vi "TermoRead.vi"() -> ()   [LabVIEW 2018]
uses:
  <vilib>/Analysis/Matrix/Datatypes/RealMatrix.ctl
  LW/Termodat_16K5/Control 2.ctl
  LW/Termodat_16K5/Control 4.ctl
  LW/Termodat_16K5/Control 3.ctl
  LW/Termodat_16K5/Control 1.ctl
  LW/Termodat_16K5/Control 5.ctl
  <instrlib>/Tektronix DMM40x0 Series/Tektronix DMM40x0 Series.lvlib
  LW/LIRA_toolbox.lvlib
  <vilib>/Analysis/Matrix/NI_Matrix.lvlib
panel:
  out "Ошибка с Modbus":errorcluster
  in  "Температура ТД":T1={"Измеряемая величина"="Ttd", "единицы измерения"="C", "Ширина строки (в символах)"="16", "Количество знаков после запятой"="2"}
  in  "Температура":T1={"Измеряемая величина"="T", "единицы измерения"="C", "Ширина строки (в символах)"="16", "Количество знаков после запятой"="2"}
  in  "Сопротивление":T1={"Измеряемая величина"="R", "единицы измерения"="Ом", "Ширина строки (в символах)"="16", "Количество знаков после запятой"="2"}
  in  "Параметры общения с Термодат":T7={"Baud Rate"=19200, "Parity"=0, "Flow Control"=0, "Timeout"=300, "Mode"=enum."RTU", "VISA resource name"="COM4", "Timeout 2"=300, "Serial Parameters"={"Mode"=enum."ASCII", "Slave Address"=1}, "Starting Address"=0, "Quantity"=1} {"Serial Parameters"."Slave Address" format="%.0x"; "Flow Control" items=["None", "XON/XOFF", "RTS/CTS", "XON/XOFF & RTS/CTS", "DTR/DSR", "XON/XOFF & DTR/DSR"]; "Parity" items=["None", "Odd", "Even", "Mark", "Space"]}
  in  "Количество датчиков Термодат":i32=2
  out "Ошибка записи в файл":errorcluster
  out "Ошибка перключения":errorcluster
  in  "Задача":refnum<k21>="Generete_Termo_Dat"
  out "T1":T8(graph)
  in  "Function (0: DC Voltage)":u16(ring)=3 items=["DC Voltage", "AC Voltage", "2 - Wire Resistance", "4 - Wire Resistance", "DC Current", "AC Current", "Frequency", "Period", "Continuity", "Diode Checking", "Temperature", "Capacitance"]
  in  "Real Matrix":T9=[[0.0, 1.0, 0.0, 0.0], [0.0, 1.0, 0.0, 0.0], [0.0, 0.0, 0.0, 1.0], [0.0, 0.0, 0.0, 1.0], [0.0, 0.0, 1.0, 1.0], [0.0, 0.0, 1.0, 1.0]]
  in  "Сопротивление при нуле":dbl=60.0
  in  "alpha":dbl=0.00428
  out "Что следует из алгоритма":bool[](array[boolean])
  out "Array":bool[][](array[boolean])
  in  "Период перключения":dbl=2.0 caption="Delay Time (s)"
  in  "Название файла":string="TempData"
  in  "Путь к файлу с указанием\n на случайный txt файл":path=path "E:/Температурные датчики/Log/20250605_19_09_TempData.txt"
  in  "Количество датчиков":i32=4
  out "Ошибка прибора":errorcluster
  out "VISA resource name out":refnum<visa-resource-name>
  out "output array":dbl[](array[numeric]) format="%^_7e"
  in  "Serial Configuration":T10={"Baud Rate"=19200, "Parity"=0, "Data Bits"=8, "Stop Bits"=10, "Flow Control"=0} {"Flow Control" items=["None", "XON/XOFF", "RTS/CTS", "XON/XOFF & RTS/CTS", "DTR/DSR", "XON/XOFF & DTR/DSR"]; "Stop Bits" items=["1.0"=10, "1.5"=15, "2.0"=20]; "Data Bits" items=["7"=7, "8"=8]; "Parity" items=["None", "Odd", "Even", "Mark", "Space"]; "Baud Rate" items=["300"=300, "600"=600, "1200"=1200, "2400"=2400, "4800"=4800, "9600"=9600, "19200"=19200]}
  in  "VISA resource name":refnum<visa-resource-name>="COM5"
  in  "stop":bool
  # "Параметры для создания log файла"
  # "Параметры для расчёта температуры"
  # "Схема включения каналов"
  # "Параметры процесса измерения"
  # "Каждая колонка соответсвует определённому датчику\nКаждый ряд соответствует определённому реле"
  # "Подключение к Tetronix DMM4040"
  # "Индикация для отадки"
  # "График температур"
  # "Параметры инициализации"
  # "Параметры чтения"
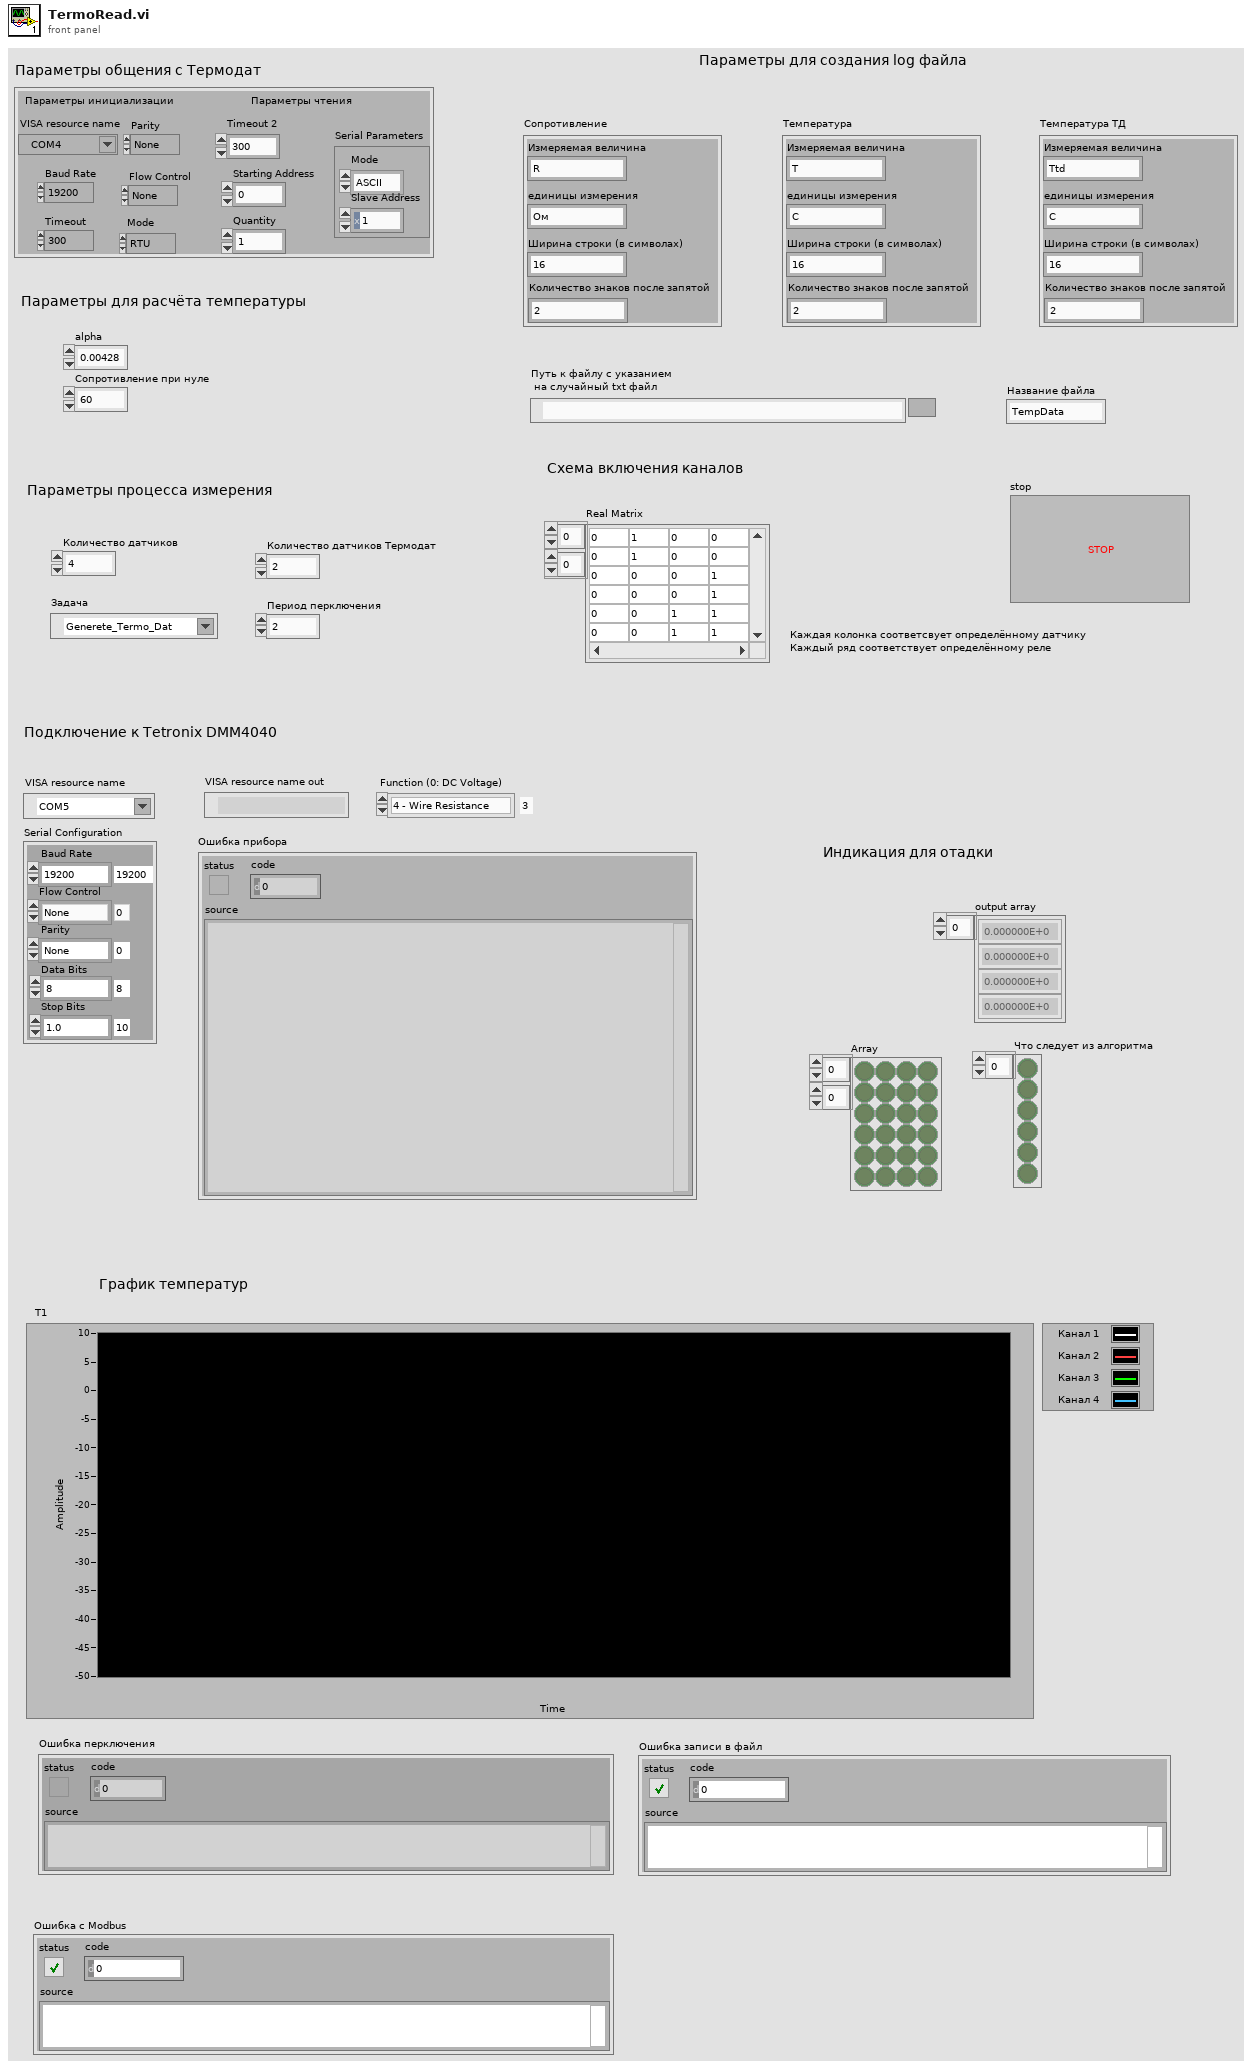
[diagram p1: front panel]
types:
  T1 = cluster{"Измеряемая величина":string, "единицы измерения":string, "Ширина строки (в символах)":string, "Количество знаков после запятой":string}
  T2 = typedef "Control 2.ctl" = u32
  T3 = typedef "Control 4.ctl" = u32
  T4 = typedef "Control 3.ctl" = enum16{"RTU", "ASCII"}
  T5 = typedef "Control 1.ctl" = refnum<visa-resource-name>
  T6 = typedef "Control 5.ctl" = u32
  T7 = cluster{"Baud Rate":T2, "Parity":u16, "Flow Control":u16, "Timeout":T3, "Mode":T4, "VISA resource name":T5, "Timeout 2":T6, "Serial Parameters":cluster{"Mode":enum16{"RTU", "ASCII"}, "Slave Address":u8}, "Starting Address":u16, "Quantity":u16}
  T8 = cluster{"Массив температур[0]":dbl, "Массив температур[1]":dbl, "Массив температур[2]":dbl, "Массив температур[3]":dbl, "Массив температур[4]":dbl, "Массив температур[5]":dbl, "Массив температур[6]":dbl, "Массив температур[7]":dbl, "Массив температур[8]":dbl}
  T9 = typedef "NI_Matrix.lvlib/RealMatrix.ctl" = dbl[][]
  T10 = cluster{"Baud Rate":u32, "Parity":u16, "Data Bits":u16, "Stop Bits":u16, "Flow Control":u16}
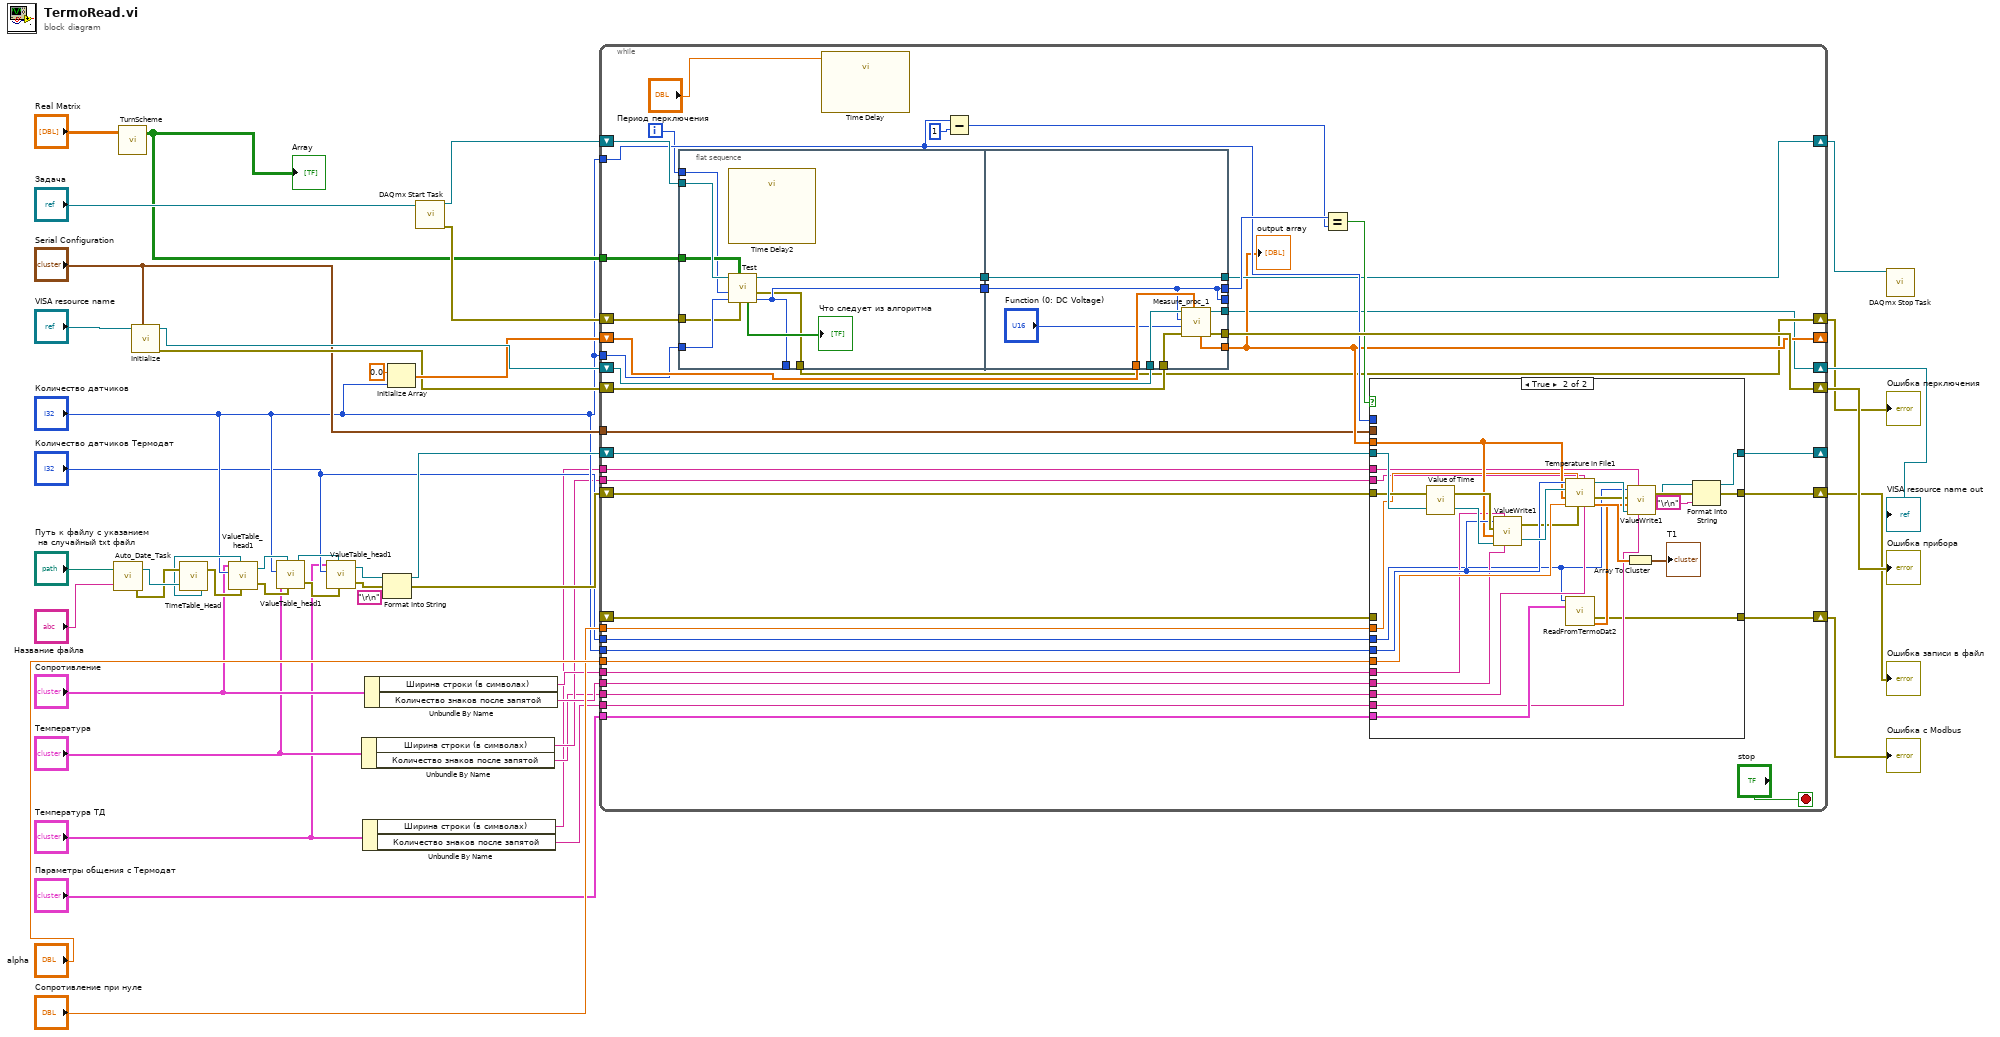
[diagram p0: block diagram]
diagram:
  n1 = call "Auto_Date_Task.vi"("Название файла"="Название файла", "Путь к файлу с указанием на случайный txt файл"="Путь к файлу с указанием\n на случайный txt файл") -> ("error out"=w27:errorcluster, "refnum out"=w33:refnum<file>)
  n2 = call "TurnScheme.vi"("Real Matrix"="Real Matrix") -> ("Array"=w22:bool[][])  [unwired: 2 in]
  "Array" <- w22
  n3 = call <instrlib>:"Initialize.vi"("Serial Configuration"="Serial Configuration", "VISA resource name"="VISA resource name") -> ("error out"=w41:errorcluster, "VISA resource name out"=w43:refnum<visa-resource-name>)  [unwired: 8 in]
  n4 = call <userlib>:"TimeTable_Head.vi"("input file"=w33, "error in"=w27) -> ("output file refnum"=w20:refnum<file>, "error out"=w19:errorcluster)
  n5 = call "ValueTable_head1.vi"("error in 2"=w19, "Файл записи"=w20, "Количество датчиков"="Количество датчиков", "Cluster"="Сопротивление") -> ("error out"=w17:errorcluster, "Файл записи 2"=w18:refnum<file>)  [unwired: 2 in]
  n6 = call "ValueTable_head1.vi"("error in 2"=w17, "Файл записи"=w18, "Количество датчиков"="Количество датчиков", "Cluster"="Температура") -> ("error out"=w14:errorcluster, "Файл записи 2"=w15:refnum<file>)  [unwired: 2 in]
  n7 = call "ValueTable_head1.vi"("error in 2"=w14, "Файл записи"=w15, "Количество датчиков"="Количество датчиков Термодат", "Cluster"="Температура ТД") -> ("error out"=w11:errorcluster, "Файл записи 2"=w12:refnum<file>)  [unwired: 2 in]
  n8 = Unbundle By Name("Температура") -> ("Ширина строки (в символах)"=w6:string, "Количество знаков после запятой"=w5:string)
  n9 = Unbundle By Name("Температура ТД") -> ("Ширина строки (в символах)"=w3:string, "Количество знаков после запятой"=w2:string)
  n10 = Unbundle By Name("Сопротивление") -> ("Ширина строки (в символах)"=w9:string, "Количество знаков после запятой"=w8:string)
  n11 = Format Into String(initial string=w12, error in=w11, "\r\n") -> (resulting string=w34:refnum<file>, error out=w26:errorcluster)  [unwired: 1 in]
  n12 = Initialize Array(0.0 ("element"), "Количество датчиков") -> (w42:dbl[])
  n13 = call <vilib>:"DAQmx Start Task.vi"("task/channels in"="Задача") -> ("task out"=w45:refnum<k21>, "error out"=w29:errorcluster)  [unwired: 13 in]
  n14 = while {
    shift-right: [w69] -> w46
    shift-left: w45 -> [w85]
    shift-right: [w80] -> w40
    shift-left: w41 -> [w81]
    tunnel: "Количество датчиков" -> [w73]
    shift-right: [w66] -> _
    shift-left: w42 -> [w79]
    shift-right: [w71] -> _
    shift-left: w34 -> [w72]
    shift-right: [w57] -> w38
    shift-left: w43 -> [w82]
    tunnel: w22 -> [w70]
    tunnel: "alpha" -> [w68]
    tunnel: "Сопротивление при нуле" -> [w67]
    tunnel: "Количество датчиков" -> [w64]
    tunnel: "Количество датчиков" -> [w63]
    shift-right: [w61] -> w28
    shift-left: w29 -> [w62]
    shift-right: [w59] -> w25
    shift-left: w26 -> [w60]
    tunnel: "Serial Configuration" -> [w58]
    tunnel: "Количество датчиков Термодат" -> [w56]
    tunnel: "Параметры общения с Термодат" -> [w55]
    tunnel: w9 -> [w54]
    tunnel: w8 -> [w53]
    tunnel: w6 -> [w52]
    tunnel: w5 -> [w51]
    tunnel: w3 -> [w50]
    tunnel: w2 -> [w49]
    shift-right: [w48] -> w1
    shift-left: _ -> [w47]
    i -> [w65]
    stop <- "stop" stop-if-true
    n15 = flat-sequence {
      tunnel: w85 -> [w127]
      tunnel: [w126] -> w84
      tunnel: [w123] -> w83
      tunnel: w70 -> [w125]
      tunnel: [w123] -> _
      tunnel: w65 -> [w122]
      tunnel: w64 -> [w121]
      tunnel: w62 -> [w120]
      tunnel: [w119] -> w61
      tunnel: w84 -> [w129]
      tunnel: w83 -> [w130]
      tunnel: w82 -> [w136]
      tunnel: [w135] -> w57
      tunnel: w81 -> [w134]
      tunnel: [w133] -> w80
      tunnel: w79 -> [w132]
      tunnel: [w131] -> w66
      tunnel: [w130] -> _
      tunnel: [w130] -> w78
      tunnel: [w129] -> w69
      frame #0 {
        n16 = call "Time Delay2"() -> ()  [unwired: 11 in, 1 out]
        n17 = call "Test.vi"("error in"=w120, "array"=w125, "Количество датчиков"=w121, "Номер иттерации"=w122, "task/channels in"=w127) -> ("Индекс переключаемого канала"=w123:i32, "error out"=w119:errorcluster, "task out"=w126:refnum<k21>, "Что следует из алгоритма"=→"Что следует из алгоритма":bool[])  [unwired: 3 in]
      }
      frame #1 {
        n18 = call "Measure_proc_1.vi"("array"=w132, "error in (no error)"=w134, "Function (0: DC Voltage)"="Function (0: DC Voltage)", "Индекс записываемого канала"=w130, "VISA resource name"=w136) -> ("error out"=w133:errorcluster, "VISA resource name out"=w135:refnum<visa-resource-name>, "output array"=w131:dbl[])  [unwired: 4 in]
      }
    }
    n19 = call "Time Delay"("Delay Time (s)"="Период перключения") -> ()  [unwired: 10 in, 1 out]
    n20 = Subtract(x=w73, y=1) -> (x-y=w76:i32)
    n21 = Equal?(x=w78, y=w76) -> (x = y?=w74:bool)
    n22 = case shown="True" w74 {
      tunnel: w73 -> [_ _]
      tunnel: w66 -> [_ w109]
      tunnel: w72 -> [w89 w116]
      tunnel: [w89 w117] -> w71
      tunnel: w68 -> [_ w108]
      tunnel: w67 -> [_ w107]
      tunnel: w63 -> [_ w110]
      tunnel: w60 -> [w88 w115]
      tunnel: [w88 w114] -> w59
      tunnel: w58 -> [_ _]
      tunnel: w56 -> [_ w90]
      tunnel: w55 -> [_ w99]
      tunnel: w54 -> [_ w97]
      tunnel: w53 -> [_ w96]
      tunnel: w52 -> [_ w95]
      tunnel: w51 -> [_ w94]
      tunnel: w50 -> [_ w93]
      tunnel: w49 -> [_ w92]
      tunnel: [w87 w91] -> w48
      tunnel: w47 -> [w87 _]
      frame False {
      }
      frame True {
        n23 = call <userlib>:"Value of Time.vi"("input file"=w116, "error in"=w115) -> ("output file refnum"=w113:refnum<file>, "error out"=w112:errorcluster)
        n24 = call "ValueWrite1.vi"("Количество знаков после запятой"=w96, "Ширина строки (в символах)"=w97, "Файл с заголовком"=w113, "Массив с измерениями"=w109, "error in"=w112, "Количество датчиков"=w110) -> ("Файл с заголовком 2"=w111:refnum<file>, "error out"=w106:errorcluster)
        n25 = call "Temperature in File1.vi"("Количество знаков после запятой"=w94, "Ширина строки (в символах)"=w95, "error in"=w106, "Сопротивление при нуле"=w107, "Значение температурного коэффициента"=w108, "массив с сопротивлениями"=w109, "Файл"=w111, "Количество датчиков"=w110) -> ("Массив температур"=w105:dbl[], "error out"=w102:errorcluster, "Файл 2"=w103:refnum<file>)  [unwired: 1 in]
        n26 = call "ReadFromTermoDat2.vi"("Количество Термодатов"=w90, "Cluster"=w99) -> ("error out"=w91:errorcluster, "output array"=w98:dbl[])  [unwired: 12 in]
        n27 = Array To Cluster(array=w105) -> (cluster=→"T1":T8)
        n28 = call "ValueWrite1.vi"("Количество знаков после запятой"=w92, "Ширина строки (в символах)"=w93, "Файл с заголовком"=w103, "Массив с измерениями"=w98, "error in"=w102, "Количество датчиков"=w90) -> ("Файл с заголовком 2"=w100:refnum<file>, "error out"=w101:errorcluster)
        n29 = Format Into String(initial string=w100, error in=w101, "\r\n") -> (resulting string=w117:refnum<file>, error out=w114:errorcluster)  [unwired: 1 in]
      }
    }
    "output array" <- w66
  }
  "VISA resource name out" <- w38
  "Ошибка прибора" <- w40
  "Ошибка перключения" <- w28
  "Ошибка записи в файл" <- w25
  "Ошибка с Modbus" <- w1
  n30 = call <vilib>:"DAQmx Stop Task.vi"("task/channels in"=w46) -> ()  [unwired: 13 in, 2 out]
